vi "RLC Series Transfer Function Magnitude in Frequency Point.vi"(8 "C, F":dbl=7.5e-06 format="%#_13g", 9 "L, H":dbl=0.01 format="%#_13g", 10 "R, Ohm":dbl=10.0 format="%#_13g", 11 "F, Hz":dbl=600.0 format="%#_13g") -> (3 "H(f)":dbl)   [LabVIEW 2019]
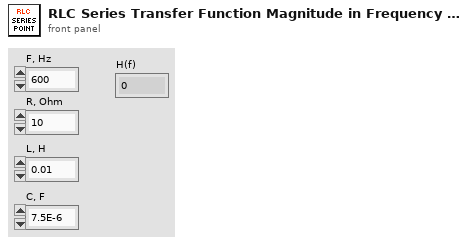
[diagram p1: front panel]
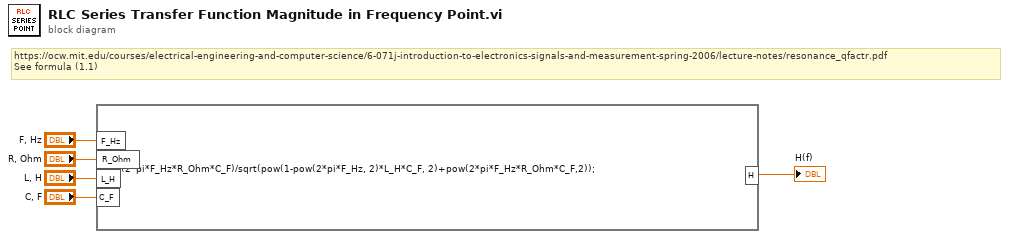
[diagram p0: block diagram]
diagram:
  # "https://ocw.mit.edu/courses/electrical-engineering-and-computer-science/6-071j-introduction-to-electronics-signals-and-measurement-spring-2006/lecture-notes/resonance_qfactr.pdf\nSee formula (1.1)"
  n1 = formula code="H=(2*pi*F_Hz*R_Ohm*C_F)/sqrt(pow(1-pow(2*pi*F_Hz, 2)*L_H*C_F, 2)+pow(2*pi*F_Hz*R_Ohm*C_F,2));"("F_Hz"="F, Hz", "R_Ohm"="R, Ohm", "L_H"="L, H", "C_F"="C, F") -> ("H"=→"H(f)":dbl)
